vi "UUTInfomation.vi"(6 "Socket:":i32, 7 "SeqModel?":bool=TRUE, 8 "error in (no error)":errorcluster, 9 "PartNumberData":T1(array[cluster]), 10 "Timeout(s)":i32, 11 "Sequence Context In":refnum<k7>) -> (0 "error out":errorcluster, 2 "Timeout":bool, 3 "Continue Testing?":bool)   [LabVIEW 2021]
doc: "Custom DUT Information dialog."
uses:
  Data/InitialStates.ctl
  Data/Data.ctl
  <vilib>/addons/TestStand/_TSUtility.llb/TestStand - Set Property Value (Boolean).vi
panel:
  out "Message":string
  in  "Barcode":string
  in  "Cancel":bool
  in  "OK":bool
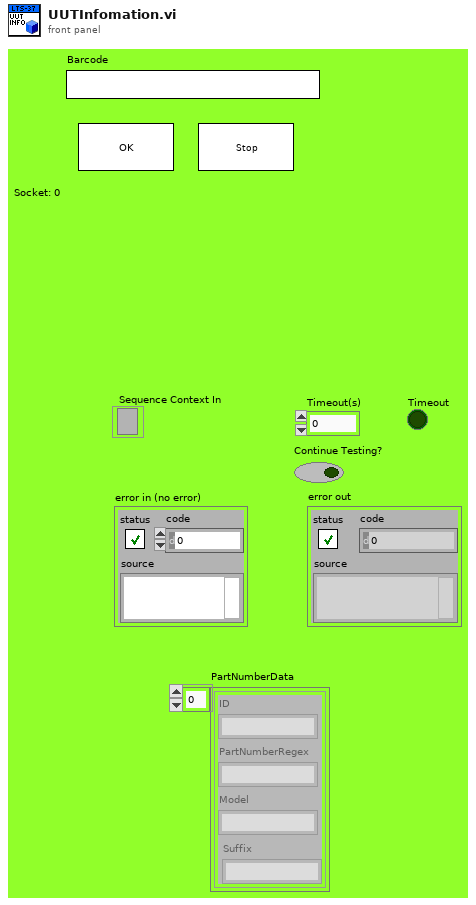
[diagram p1: front panel]
types:
  T1 = cluster{"ID":string, "PartNumberRegex":string, "Model":string, "Suffix":string}[]
  T2 = typedef "Data.ctl" = cluster{"ThisVIref":refnum<vi>, "PnlRef":refnum<vi>, "PartNumberData":cluster{"ID":string, "PartNumberRegex":string, "Model":string, "Suffix":string}[], "Timeout":bool, "ContinueTesting?":bool, "isInitialLogIn":bool, "Timeout(ms)":i32}
  T3 = typedef "InitialStates.ctl" = enum16{"Initialize", "Find Regex", "Wait For Event", "Exit"}
  T4 = typedef "TestStand - Status Monitor.ctl" = cluster{"Sequence Context":refnum<k7>, "Execution":refnum<k7>, "Termination Monitor":refnum<k7>}
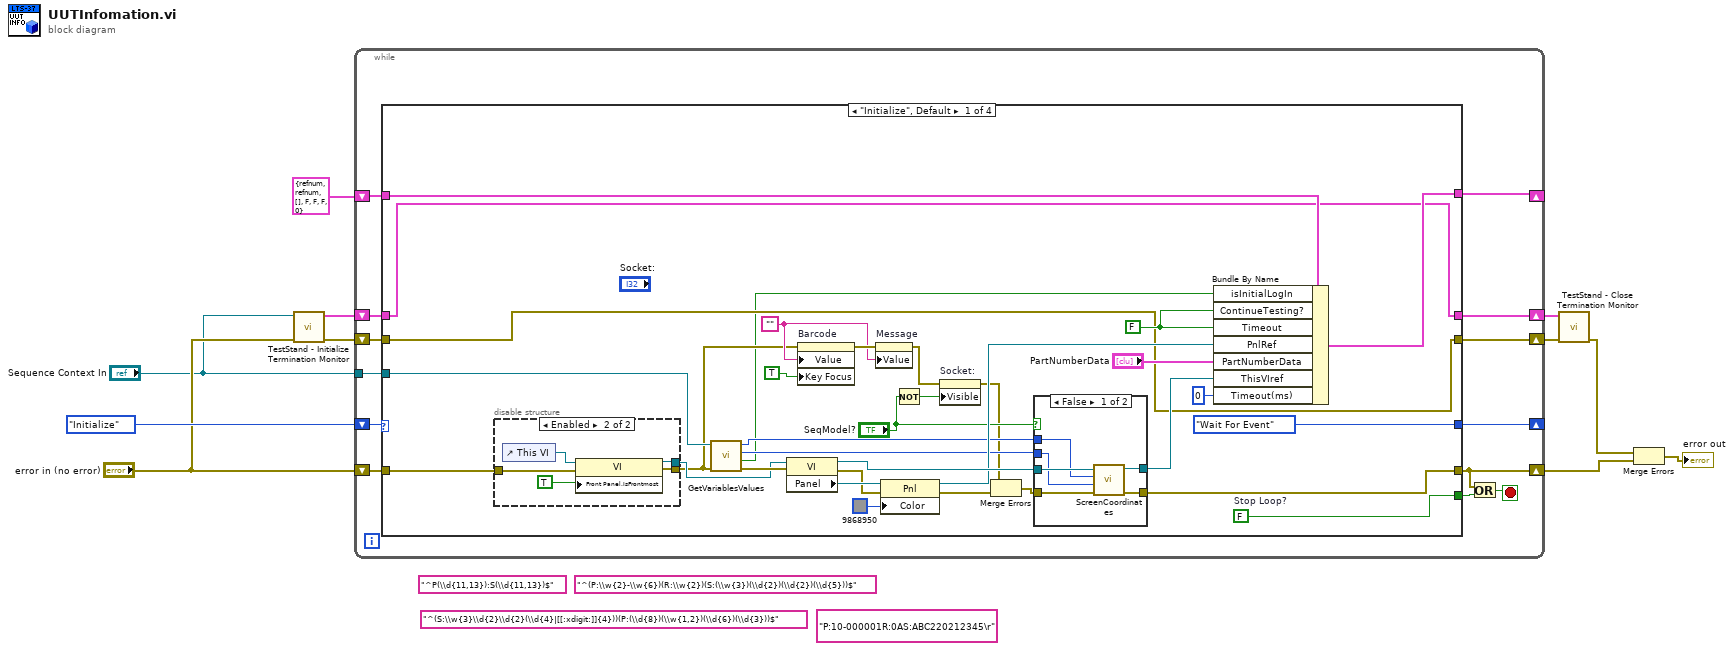
[diagram p0: block diagram]
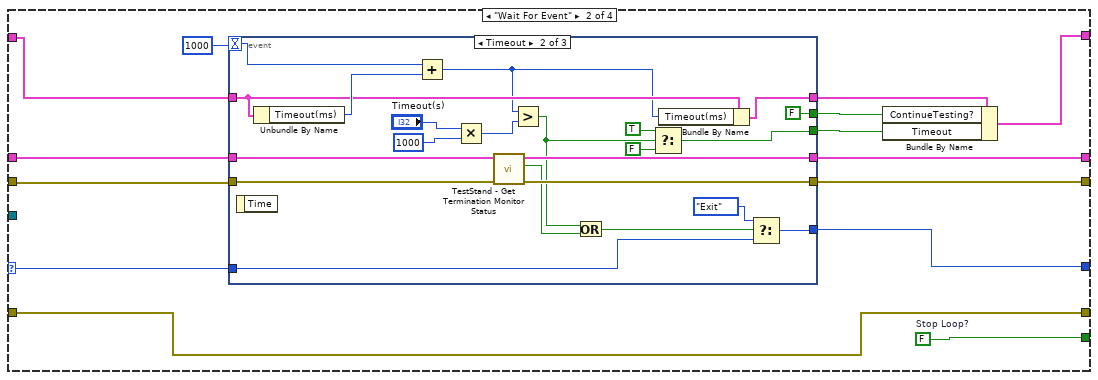
[diagram p4: hidden frame]
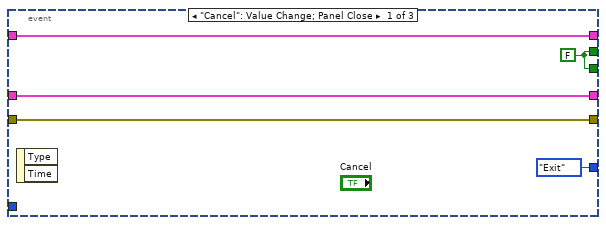
[diagram p5: hidden frame]
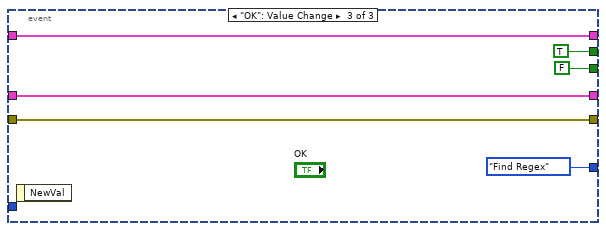
[diagram p6: hidden frame]
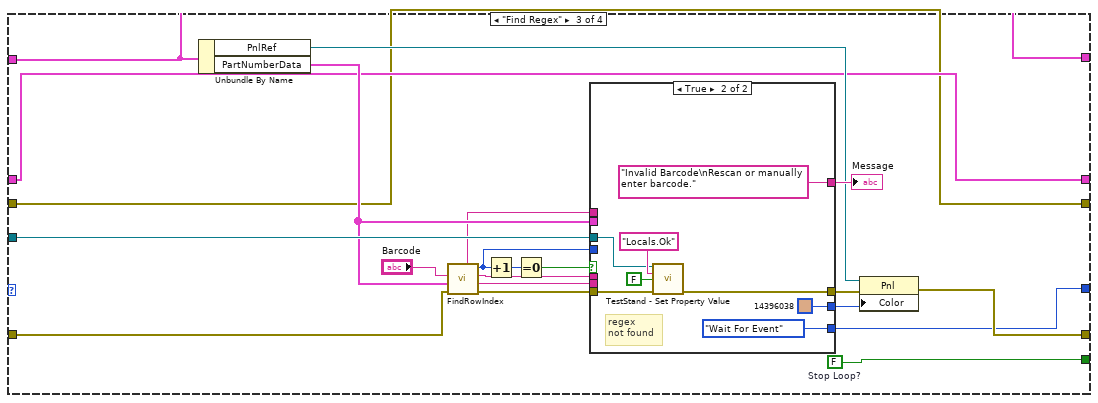
[diagram p7: hidden frame]
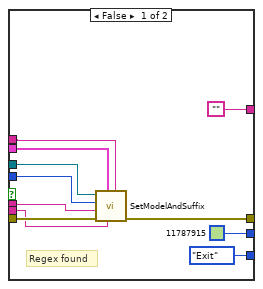
[diagram p8: hidden frame]
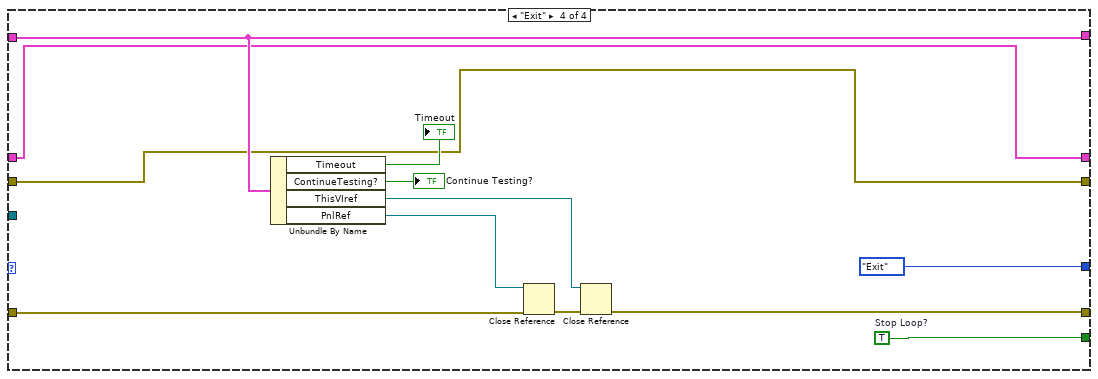
[diagram p9: hidden frame]
diagram:
  (unwired) "P:10-000001R:0AS:ABC220212345\r"
  (unwired) "^(P:\\w{2}-\\w{6})(R:\\w{2})(S:(\\w{3})(\\d{2})(\\d{2})(\\d{5}))$"
  (unwired) "^(S:\\w{3}\\d{2}\\d{2}(\\d{4}|[[:xdigit:]]{4}))(P:(\\d{8})(\\w{1,2})(\\d{6})(\\d{3}))$"
  (unwired) "^P(\\d{11,13}):S(\\d{11,13})$" ("regular expression")
  n1 = call <vilib>:"TestStand - Initialize Termination Monitor.vi"("error in (no error)"="error in (no error)", "Sequence Context In"="Sequence Context In") -> ("error out"=w4:errorcluster, "Status Monitor Out"=w5:T4)  [unwired: 8 in]
  n2 = while {
    shift-right: [w19] -> _
    shift-left: InitialStates."Initialize" -> [w24]
    shift-right: [w20] -> _
    shift-left: T2 {"ThisVIref"=refnum, "PnlRef"=refnum, "PartNumberData"=[], "Timeout"=FALSE, "ContinueTesting?"=FALSE, "isInitialLogIn"=FALSE, "Timeout(ms)"=0} ("Data") -> [w23]
    tunnel: "Sequence Context In" -> [w22]
    shift-right: [w18] -> w8
    shift-left: "error in (no error)" -> [w21]
    shift-right: [w12] -> w2
    shift-left: w5 -> [w15]
    shift-right: [w13] -> w3
    shift-left: w4 -> [w14]
    stop <- w16 stop-if-true
    n3 = case shown="\"Initialize\", Default" w24 {
      selector: w24 -> [_ w73 _ _]
      tunnel: w23 -> [w51 w84 w120 w168]
      tunnel: w22 -> [w39 _ w132 _]
      tunnel: w21 -> [w28 w83 w135 w163]
      tunnel: [w49 w80 w120 w168] -> w20
      tunnel: [InitialStates."Wait For Event" w85 w127 InitialStates."Exit"] -> w19
      tunnel: [w35 w83 w133 w159] -> w18
      tunnel: [w47 w82 w126 w162] -> w17
      tunnel: w15 -> [w38 w76 w122 w161]
      tunnel: w14 -> [w37 w72 w121 w160]
      tunnel: [w37 w75 w121 w160] -> w13
      tunnel: [w38 w74 w122 w161] -> w12
      frame "Initialize", Default {
        w42 = FALSE ("Timeout")
        w47 = FALSE  # Stop Loop?
        w53 = ""
        n4 = disable-structure shown="Enabled" {
          disable-tunnel: w28 -> [w58 w62]
          disable-tunnel: [w58 w61] -> w27
          disable-tunnel: [_ w60] -> w40
          frame Disabled {
          }
          frame Enabled {
            n5 = control-ref of="This VI"() -> (w63:refnum<vi>)
            n6 = property class="VI"(reference=w63, error in=w62, "Front Panel.IsFrontmost"=TRUE ("Front Panel Window:Is Frontmost")) -> (reference out=w60:refnum<vi>, error out=w61:errorcluster)
          }
        }
        n7 = call "GetVariablesValues .vi"("error in (no error)"=w27, "Sequence Context In"=w39) -> ("error out (no error)"=w41:errorcluster, "isInitialLogIn"=w25:bool, "LeftCoordinates"=w45:i16, "TopCoordinates"=w46:i16)  [unwired: 6 in]
        n8 = property class="VI"(reference=w40, error in=w41) -> (reference out=w52:refnum<vi>, error out=w55:errorcluster, "Panel"=w56:refnum<vi>)
        n9 = property on="Barcode" class="Str"(error in=w27, "Value"=w53, "Key Focus"=TRUE) -> (error out=w54:errorcluster)  [unwired: 1 in, 1 out]
        n10 = property on="Message" class="Str"(error in=w54, "Value"=w53) -> (error out=w33:errorcluster)  [unwired: 1 in, 1 out]
        n11 = property class="Pnl"(reference=w56, error in=w55, "Color"=u32 9868950 ("Color Box")) -> (reference out=w50:refnum<vi>, error out=w34:errorcluster)
        n12 = Not(x="SeqModel?") -> (.not. x?=w31:bool)
        n13 = property on="Socket:" class="DigNum (strict)"(error in=w33, "Visible"=w31) -> (error out=w29:errorcluster)  [unwired: 1 in, 1 out]
        n14 = Merge Errors(w29, w34) -> (w30:errorcluster)
        n15 = case shown="False" "SeqModel?" {
          tunnel: w30 -> [w69 w71]
          tunnel: [w68 w71] -> w35
          tunnel: w52 -> [w67 w70]
          tunnel: w46 -> [w66 _]
          tunnel: w45 -> [w65 _]
          tunnel: [w64 w70] -> w43
          frame False {
            n16 = call "ScreenCoordinates.vi"("error in (no error)"=w69, "Left Coordinate"=w65, "Top Coordinate"=w66, "ThisVI"=w67) -> ("error out"=w68:errorcluster, "reference out"=w64:refnum<vi>)  [unwired: 6 in]
          }
          frame True {
          }
        }
        n17 = Bundle By Name(cluster=w51, "isInitialLogIn"=w25, "ContinueTesting?"=w42, "Timeout"=w42, "PnlRef"=w50, "PartNumberData"="PartNumberData", "ThisVIref"=w43, "Timeout(ms)"=0) -> (w49:T2)
      }
      frame "Wait For Event" {
        w82 = FALSE  # Stop Loop?
        n18 = event shown="[1] Timeout" {
          selector: _ -> [_ _ _]
          dyn-events: _ -> [_ _ _]
          timeout: 1000 -> [_ w106 _]
          tunnel: [InitialStates."Exit" w94 InitialStates."Find Regex"] -> w85
          tunnel: [w89 w101 w117] -> w81
          tunnel: w84 -> [w89 w103 w117]
          tunnel: [w88 FALSE TRUE] -> w79
          tunnel: [w88 w95 FALSE ("Timeout")] -> w78
          tunnel: w76 -> [w87 w112 w114]
          tunnel: w72 -> [w86 w111 w113]
          tunnel: [w86 w110 w113] -> w75
          tunnel: [w87 w109 w114] -> w74
          tunnel: w73 -> [_ w107 _]
          event "Cancel": Value Change; Panel Close {
            w88 = FALSE
            n19 = event-data() -> ()  [unwired: 1 in, 2 out]
          }
          event Timeout {
            n20 = event-data() -> ()  [unwired: 1 in, 1 out]
            n21 = Unbundle By Name(w103) -> ("Timeout(ms)"=w104:i32)
            n22 = Add(x=w106, y=w104) -> (x+y=w102:i32)
            n23 = Multiply(x="Timeout(s)", y=1000) -> (x*y=w100:i32)
            n24 = call <vilib>:"TestStand - Get Termination Monitor Status.vi"("error in (no error)"=w111, "Status Monitor In"=w112) -> ("error out"=w110:errorcluster, "Terminating or Aborting"=w98:bool, "Status Monitor Out"=w109:T4)  [unwired: 7 in]
            n25 = Greater?(x=w102, y=w100) -> (0:w91:bool)
            n26 = Or(x=w91, y=w98) -> (x .or. y?=w93:bool)
            n27 = Select(t=TRUE ("Timeout"), s=w91, f=FALSE) -> (s? t:f=w95:bool)
            n28 = Bundle By Name(cluster=w103, "Timeout(ms)"=w102) -> (w101:T2)
            n29 = Select(t=InitialStates."Exit", s=w93, f=w107) -> (s? t:f=w94:T3)
          }
          event "OK": Value Change {
            n30 = event-data() -> ()  [unwired: 1 in, 1 out]
          }
        }
        n31 = Bundle By Name(cluster=w81, "ContinueTesting?"=w79, "Timeout"=w78) -> (w80:T2)
      }
      frame "Find Regex" {
        w126 = FALSE  # Stop Loop?
        n32 = Unbundle By Name(w120) -> ("PnlRef"=w136:refnum<vi>, "PartNumberData"=w125:T1)
        n33 = call "FindRowIndex.vi"("error in (no error)"=w135, "PartNumberData"=w125, "Barcode"="Barcode") -> ("error out"=w129:errorcluster, "SerialNumber"=w123:string, "PartNumber"=w124:string, "ArrayIndex"=w131:i32, "Revision"=w119:string)  [unwired: 4 in]
        n34 = Increment(x=w131) -> (x+1=w139:i32)
        n35 = Equal To 0?(x=w139) -> (x = 0?=w138:bool)
        n36 = case shown="True" w138 {
          tunnel: ["" "Invalid Barcode\nRescan or manually enter barcode." ("message")] -> w137
          tunnel: [u32 11787915 ("Color Box") u32 14396038 ("Color Box")] -> w134
          tunnel: w132 -> [w146 w153]
          tunnel: w131 -> [w145 _]
          tunnel: w125 -> [w143 _]
          tunnel: w129 -> [w148 w154]
          tunnel: [w147 w152] -> w128
          tunnel: [InitialStates."Exit" InitialStates."Wait For Event"] -> w127
          tunnel: w124 -> [w142 _]
          tunnel: w123 -> [w141 _]
          tunnel: w119 -> [w140 _]
          frame False {
            # "Regex found"
            n37 = call "SetModelAndSuffix.vi"("Revision"=w140, "Serial Number"=w141, "PartNumberData"=w143, "error in (no error)"=w148, "Part Number"=w142, "ArrayIndex"=w145, "Sequence Context In"=w146) -> ("error out"=w147:errorcluster)  [unwired: 3 in, 1 out]
          }
          frame True {
            # "regex \nnot found"
            n38 = call-poly <vilib>:"TestStand - Set Property Value.vi"("Sequence Context In"=w153, "Lookup String"="Locals.Ok", "New Value"=FALSE, "error in (no error)"=w154) -> ("error out"=w152:errorcluster)  [unwired: 10 in, 1 out]
          }
        }
        "Message" <- w137
        n39 = property class="Pnl"(reference=w136, error in=w128, "Color"=w134) -> (error out=w133:errorcluster)  [unwired: 1 out]
      }
      frame "Exit" {
        w162 = TRUE  # Stop Loop?
        n40 = Unbundle By Name(w168) -> ("Timeout"=→"Timeout":bool, "ContinueTesting?"=→"Continue Testing?":bool, "ThisVIref"=w166:refnum<vi>, "PnlRef"=w167:refnum<vi>)
        n41 = Close Reference(reference=w167, error in (no error)=w163) -> (error out=w169:errorcluster)
        n42 = Close Reference(reference=w166, error in (no error)=w169) -> (error out=w159:errorcluster)
      }
    }
    n43 = Or(x=w18, y=w17) -> (x .or. y?=w16:bool)
  }
  n44 = call <vilib>:"TestStand - Close Termination Monitor.vi"("error in (no error)"=w3, "Status Monitor In"=w2) -> ("error out"=w1:errorcluster)  [unwired: 9 in]
  n45 = Merge Errors(w1, w8) -> (→"error out":errorcluster)
